vi "rs3 init api.vi"(8 "error in (no error)":errorcluster) -> (0 "error out":errorcluster, 1 "Init API error":string="No Error\rNo Error", 2 "rscontext":u64=1752067024, 3 "api_version":i32=20710)   [LabVIEW 2017, in "libRealSense3.lvlib"]
doc: "Initialized communication to the RealSense API. \n\nReturns:\nError Error text\nrscontext Context handle that needs to be used in INIT ALL\napi version The libRS API version number"
uses:
  libRealSense3.lvlib
panel:
  # "RS3 Init API"
  # "(C) 2017 Intel Corp.,  AGJ"
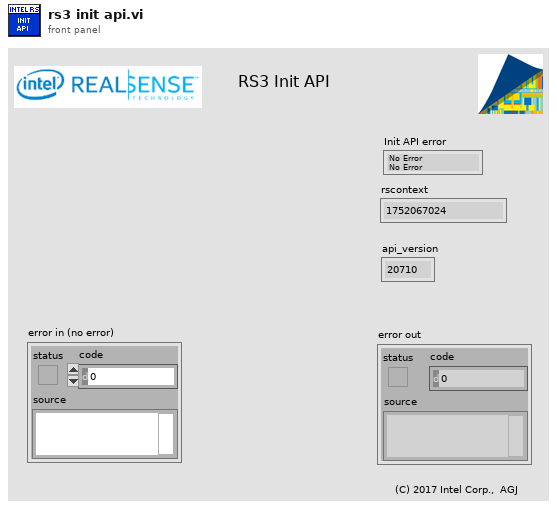
[diagram p1: front panel]
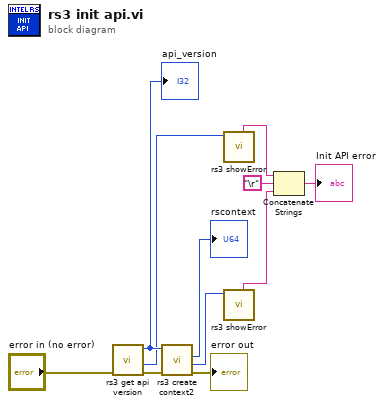
[diagram p0: block diagram]
diagram:
  n1 = call "rs3 get api version.vi"("error in (no error)"="error in (no error)") -> ("error out"=w10:errorcluster, "error"=w5:u64, "api_version"=w11:i32)  [unwired: 8 in]
  "api_version" <- w11
  n2 = call "rs3 create context2.vi"("error in (no error)"=w10, "api_version"=w11) -> ("error out"=→"error out":errorcluster, "error"=w6:u64, "rscontext"=→"rscontext":u64)  [unwired: 7 in]
  n3 = call "rs3 showError.vi"("error"=w5) -> ("Error summary"=w4:string)  [unwired: 6 in, 4 out]
  n4 = call "rs3 showError.vi"("error"=w6) -> ("Error summary"=w2:string)  [unwired: 6 in, 4 out]
  n5 = Concatenate Strings(w4, "\r", w2) -> (→"Init API error":string)
